vi "MulticolumnListbox.vi"(0 "Multicolumn Listbox":i32(listbox)) -> ()   [LabVIEW 2020]
uses:
  <vilib>/Utility/miscctls.llb/LVRowAndColumnTypeDef.ctl
panel:
  out "error out":errorcluster
  in  "error in (no error)":errorcluster
  # "Hover a particular row header to get that header\nhighlighted and double-click particukar row to provide\nvalues and click enter to accept the value."
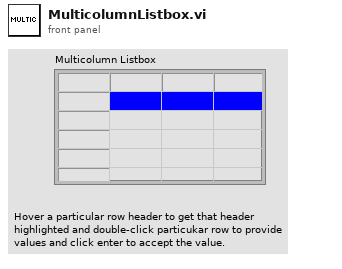
[diagram p1: front panel]
types:
  T1 = typedef "LVRowAndColumnTypeDef.ctl" = cluster{"Row":i32, "Column":i32}
  T2 = typedef "LVPoint32TypeDef.ctl" = cluster{"Horizontal":i32, "Vertical":i32}
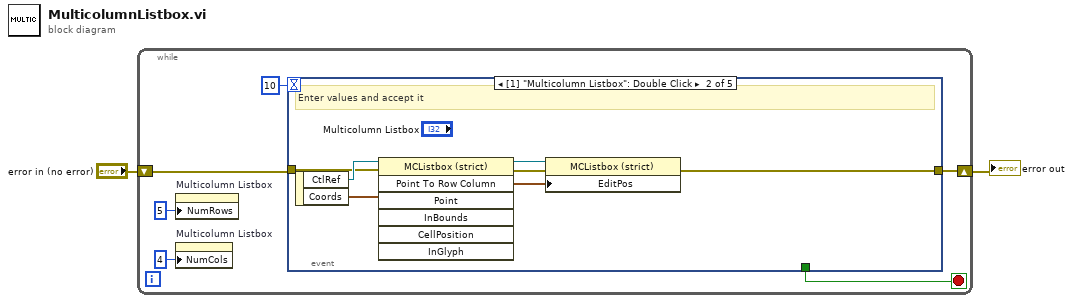
[diagram p0: block diagram]
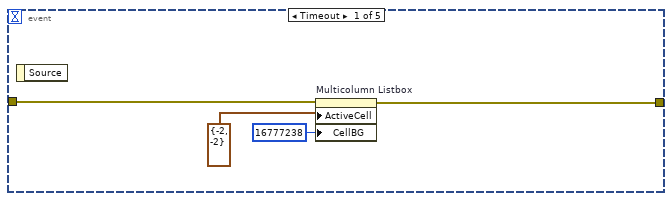
[diagram p2: hidden frame]
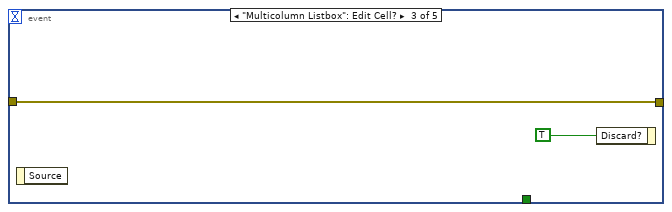
[diagram p3: hidden frame]
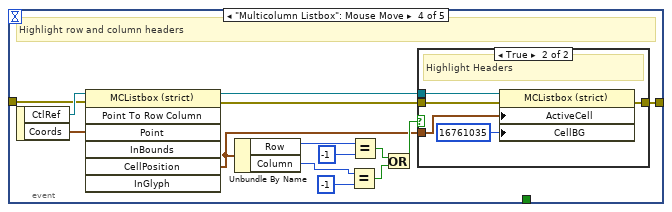
[diagram p4: hidden frame]
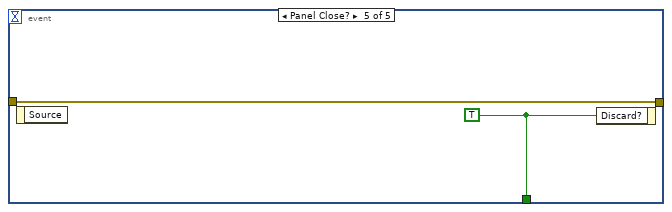
[diagram p6: hidden frame]
diagram:
  n1 = while {
    shift-right: [w8] -> w1
    shift-left: "error in (no error)" -> [w7]
    stop <- w6 stop-if-true
    n2 = property on="Multicolumn Listbox" class="MCListbox (strict)"("NumRows"=u32 5 ("Number of Rows")) -> ()  [unwired: 2 in, 2 out]
    n3 = property on="Multicolumn Listbox" class="MCListbox (strict)"("NumCols"=u32 4 ("Number of Columns")) -> ()  [unwired: 2 in, 2 out]
    n4 = event shown="[1] \"Multicolumn Listbox\": Double Click" {
      selector: _ -> [_ _ _ _ _]
      dyn-events: _ -> [_ _ _ _ _]
      timeout: 10 -> [_ _ _ _ _]
      tunnel: [w12 w13 w20 w25 w42] -> w8
      tunnel: w7 -> [w11 w16 w20 w34 w42]
      tunnel: [_ _ _ _ w43] -> w6
      event Timeout {
        n5 = event-data() -> ()  [unwired: 1 in, 1 out]
        n6 = property on="Multicolumn Listbox" class="MCListbox (strict)"(error in=w11, "ActiveCell"=T1 {"Row"=-2, "Column"=-2} ("Active Cell:Active Cell"), "CellBG"=u32 16777238 ("Active Cell:Cell Background Color")) -> (error out=w12:errorcluster)  [unwired: 1 in, 1 out]
      }
      event "Multicolumn Listbox": Double Click {
        # "Enter values and accept it"
        n7 = event-data() -> ("CtlRef"=w19:refnum<vi>, "Coords"=w15:T2)  [unwired: 1 in]
        n8 = invoke class="MCListbox (strict)" method="Point To Row Column"(reference=w19, error in=w16, "Point"=w15) -> (reference out=w17:refnum<vi>, error out=w18:errorcluster, "CellPosition"=w14:T1)  [unwired: 4 in, 4 out]
        n9 = property class="MCListbox (strict)"(reference=w17, error in=w18, "EditPos"=w14) -> (error out=w13:errorcluster)  [unwired: 1 out]
      }
      event "Multicolumn Listbox": Edit Cell? {
        n10 = event-data() -> ()  [unwired: 1 in, 1 out]
        n11 = event-data("Discard?"=TRUE) -> ()  [unwired: 1 in, 1 out]
      }
      event "Multicolumn Listbox": Mouse Move {
        # "Highlight row and column headers"
        n12 = event-data() -> ("CtlRef"=w35:refnum<vi>, "Coords"=w33:T2)  [unwired: 1 in]
        n13 = invoke class="MCListbox (strict)" method="Point To Row Column"(reference=w35, error in=w34, "Point"=w33) -> (reference out=w23:refnum<vi>, error out=w22:errorcluster, "CellPosition"=w24:T1)  [unwired: 4 in, 4 out]
        n14 = Unbundle By Name(w24) -> ("Row"=w32:i32, "Column"=w29:i32)
        n15 = Equal?(x=w29, y=-1) -> (x = y?=w27:bool)
        n16 = Equal?(x=w32, y=-1) -> (x = y?=w28:bool)
        n17 = Or(x=w28, y=w27) -> (x .or. y?=w26:bool)
        n18 = case shown="True" w26 {
          tunnel: w23 -> [_ w41]
          tunnel: w22 -> [w36 w39]
          tunnel: [w36 w38] -> w25
          tunnel: w24 -> [_ w37]
          frame False {
          }
          frame True {
            # "Highlight Headers"
            n19 = property class="MCListbox (strict)"(reference=w41, error in=w39, "ActiveCell"=w37, "CellBG"=u32 16761035 ("Active Cell:Cell Background Color")) -> (error out=w38:errorcluster)  [unwired: 1 out]
          }
        }
      }
      event Panel Close? {
        w43 = TRUE ("Discard?")
        n20 = event-data() -> ()  [unwired: 1 in, 1 out]
        n21 = event-data("Discard?"=w43) -> ()  [unwired: 1 in, 1 out]
      }
    }
  }
  "error out" <- w1
